vi "(SubVI) Fixed-Window Median Filters_YCC.vi"(5 "Avg points":i32, 7 "Signal":dbl[](array[numeric])) -> (3 "Filtered Signal":dbl[](array[numeric]))   [LabVIEW 2014]
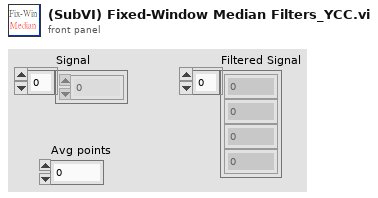
[diagram p1: front panel]
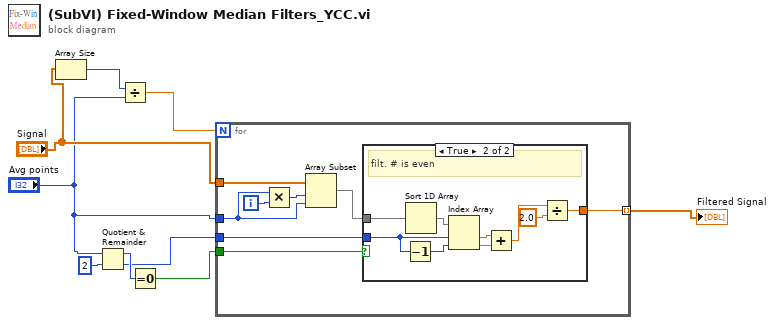
[diagram p0: block diagram]
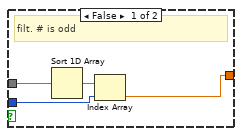
[diagram p2: hidden frame]
diagram:
  n1 = Array Size(array="Signal") -> (size(s)=w3:i32)
  n2 = Quotient & Remainder(x="Avg points", y=2) -> (x-y*floor(x/y)=w9:i32, floor(x/y)=w6:i32)
  n3 = Divide(x=w3, y="Avg points") -> (x/y=w1:dbl)
  n4 = Equal To 0?(x=w9) -> (x = 0?=w7:bool)
  n5 = for {
    N: w1 -> [_]
    tunnel: "Signal" -> [w16]
    tunnel: w7 -> [w17]
    tunnel: "Avg points" -> [w12]
    tunnel: w6 -> [w11]
    tunnel: [w10] -> w5 mode=indexing
    i -> [w15]
    n6 = Multiply(x=w12, y=w15) -> (x*y=w14:i32)
    n7 = Array Subset(array=w16, index=w14, length=w12) -> (w13:dbl[])
    n8 = case shown="True" w17 {
      tunnel: w13 -> [w20 w30]
      tunnel: w11 -> [w19 w28]
      tunnel: [w18 w22] -> w10
      frame False {
        # "filt. # is odd"
        n9 = Sort 1D Array(array=w20) -> (sorted array=w21:dbl[])
        n10 = Index Array(array=w21, index=w19) -> (element=w18:dbl)
      }
      frame True {
        # "filt. # is even"
        n11 = Decrement(x=w28) -> (x-1=w27:i32)
        n12 = Sort 1D Array(array=w30) -> (sorted array=w29:dbl[])
        n13 = Index Array(array=w29, index #1=w28, index #2=w27) -> (element #1=w26:dbl, element #2=w25:dbl)
        n14 = Add(x=w26, y=w25) -> (x+y=w24:dbl)
        n15 = Divide(x=w24, y=2.0) -> (x/y=w22:dbl)
      }
    }
  }
  "Filtered Signal" <- w5
